vi "ingresaMediciones.vi"(8 "error in (no error)":errorcluster, 9 "Tbl Refnum":refnum<vi>, 10 "New Value":string[][](array[string]), 11 "Prueba07 in":refnum<class "Prueba07.lvclass">) -> (0 "error out":errorcluster, 3 "Prueba07 out":refnum<class "Prueba07.lvclass">)   [LabVIEW 2019, in "Prueba07.lvclass"]
uses:
  Prueba07.lvclass
  Prueba07.lvclass/Prueba07.ctl
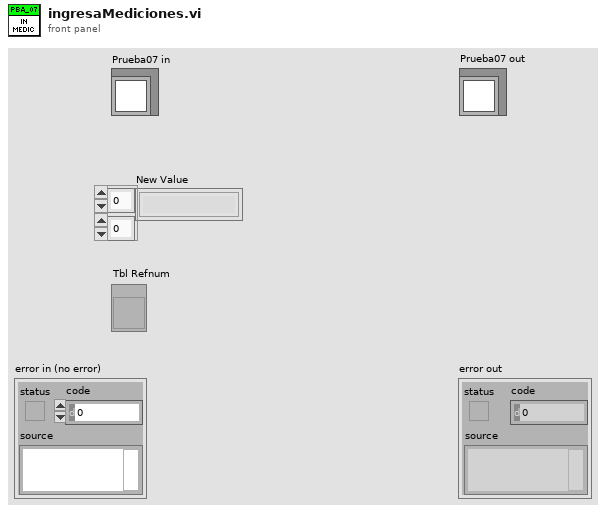
[diagram p1: front panel]
types:
  T1 = cluster{"Medido":dbl, "Error":dbl, "Ref":dbl, "Incert_exp":dbl, "Tol+":dbl, "Tol-":dbl, "fila":i32}
  T2 = typedef "LVRowAndColumnTypeDef.ctl" = cluster{"Row":i32, "Column":i32}
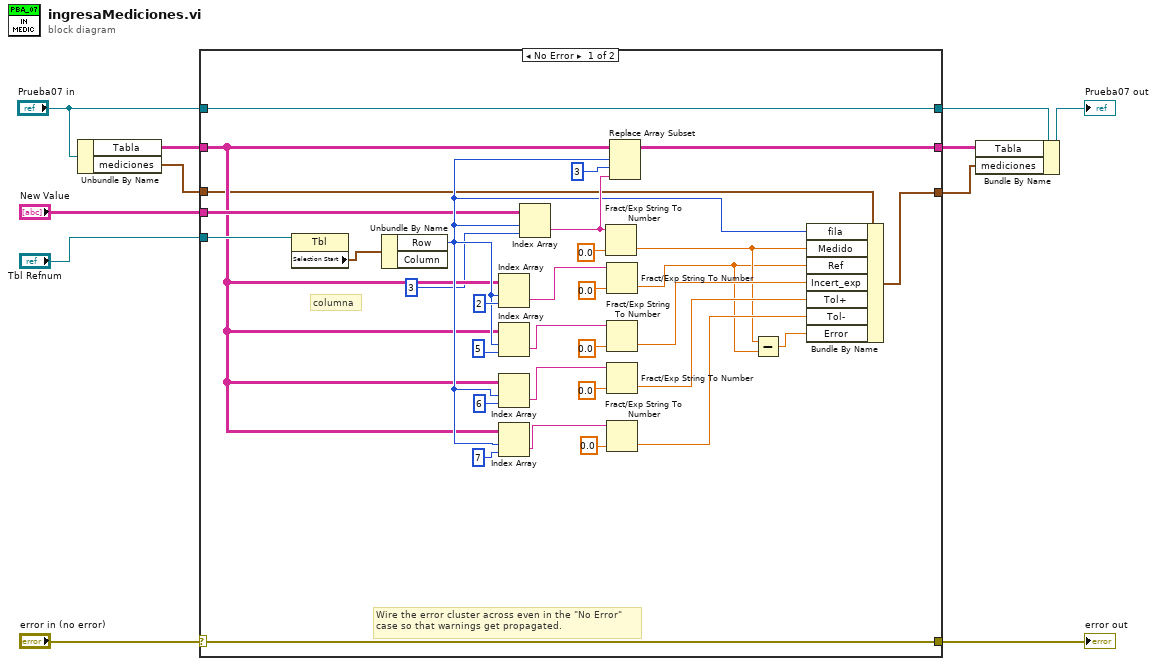
[diagram p0: block diagram]
diagram:
  n1 = Unbundle By Name("Prueba07 in") -> ("Tabla"=w5:string[][], "mediciones"=w4:T1)
  n2 = case shown="No Error" "error in (no error)" {
    selector: "error in (no error)" -> [w42 w47]
    tunnel: [w42 w47] -> w10
    tunnel: [w43 w46] -> w9
    tunnel: "Prueba07 in" -> [w43 w46]
    tunnel: w5 -> [w19 w45]
    tunnel: "New Value" -> [w22 _]
    tunnel: "Tbl Refnum" -> [w21 _]
    tunnel: w4 -> [w18 w44]
    tunnel: [w17 w45] -> w2
    tunnel: [w16 w44] -> w1
    frame No Error {
      # "columna"
      # "Wire the error cluster across even in the \"No Error\"\ncase so that warnings get propagated."
      n3 = property on="Property Node" class="Tbl"(reference=w21) -> ("Selection Start"=w20:T2)  [unwired: 1 in, 2 out]
      n4 = Unbundle By Name(w20) -> ("Row"=w23:i32)  [unwired: 1 out]
      n5 = Index Array(array=w19, index (row)=w23, index (col)=2 ("disabled index (col)")) -> (element=w38:string)
      n6 = Index Array(array=w19, index (row)=w23, index (col)=5 ("index (row)")) -> (element=w34:string)
      n7 = Index Array(array=w19, index (row)=w23, index (col)=6 ("disabled index (col)")) -> (element=w25:string)
      n8 = Index Array(array=w19, index (row)=w23, index (col)=7 ("index (row)")) -> (element=w28:string)
      n9 = Index Array(array=w22, index (row)=w23, index (col)=3) -> (element=w24:string)
      n10 = Fract/Exp String To Number(string=w24, default (0 dbl)=0.0) -> (number=w15:dbl)  [unwired: 2 in, 1 out]
      n11 = Fract/Exp String To Number(string=w38, default (0 dbl)=0.0) -> (number=w14:dbl)  [unwired: 2 in, 1 out]
      n12 = Fract/Exp String To Number(string=w34, default (0 dbl)=0.0) -> (number=w33:dbl)  [unwired: 2 in, 1 out]
      n13 = Fract/Exp String To Number(string=w25, default (0 dbl)=0.0) -> (number=w26:dbl)  [unwired: 2 in, 1 out]
      n14 = Fract/Exp String To Number(string=w28, default (0 dbl)=0.0) -> (number=w27:dbl)  [unwired: 2 in, 1 out]
      n15 = Replace Array Subset(array=w19, new element=w24, index (row)=w23, index (col)=3 ("disabled index (col)")) -> (w17:string[][])
      n16 = Subtract(x=w15, y=w14) -> (x-y=w13:dbl)
      n17 = Bundle By Name(cluster=w18, "fila"=w23, "Medido"=w15, "Ref"=w14, "Incert_exp"=w33, "Tol+"=w26, "Tol-"=w27, "Error"=w13) -> (w16:T1)
    }
    frame Error {
    }
  }
  "error out" <- w10
  n18 = Bundle By Name(cluster=w9, "Tabla"=w2, "mediciones"=w1) -> (→"Prueba07 out":refnum<class "Prueba07.lvclass">)
